vi "PositionToRollTatic.vi"(7 "Game in":refnum<class "Game.lvclass">, 8 "error in (no error)":errorcluster, 9 "first call":bool, 10 "Robot":refnum<class "Robot.lvclass">, 11 "PositionToRollTatic in":refnum<class "PositionToRollTatic.lvclass">) -> (0 "error out":errorcluster, 2 "Robot out":refnum<class "Robot.lvclass">, 3 "PositionToRollTatic out":refnum<class "PositionToRollTatic.lvclass">)   [LabVIEW 2018, in "PositionToRollTatic.lvclass"]
uses:
  PositionToRollTatic.lvclass
  Robot_class/Robot.lvclass
  Game_class/Game.lvclass
  Tactic_class/Tactic.lvclass/Tactic.ctl
  Robot_class/tactics.ctl
  Skillbook_class/Skillbook.lvclass/Skillbook.ctl
  Object_class/Object.lvclass/Object.ctl
  Robot_class/Robot.lvclass/Robot.ctl
  <vilib>/Analysis/_algsub.llb/Real Vector Norm.vi
  Skillbook_class/Read PositionToRollSkill.vi
  Object_class/Read x.vi
  Object_class/Read y.vi
  Robot_class/Read orientation.vi
  Robot_class/Read dest_x.vi
  Robot_class/Read dest_y.vi
  Robot_class/Read dest_orientation.vi
  Skillbook_class/Read HaltSkill.vi
  Tactic_class/Read Skillbook.vi
  Robot_class/Write tactic.vi
  Skillbook_class/Skillbook.lvclass
  PositionToRollSkill_class/PositionToRollSkill.lvclass
  HaltSkill_class/HaltSkill.lvclass
  <vilib>/Analysis/NI_AALPro.lvlib
panel:
  out "Sucsses":bool
  out "x .or. y?":bool
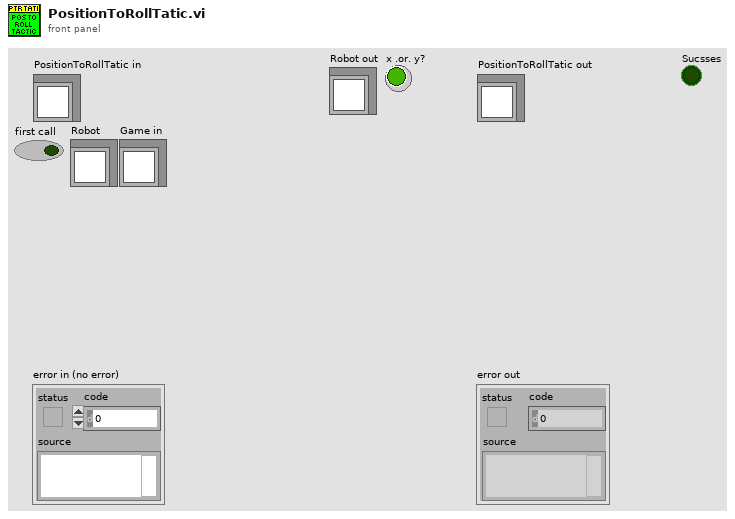
[diagram p1: front panel]
types:
  T1 = typedef "tactics.ctl" = enum16{"Roller", "PrepareRollToPassRollerGoTo", "PrepareRollToPassReceiverGoTo", "WaitRoll", "PositionToRoll", "PenaltyAttacker", "PassObserver", "PenaltyDefense", "Test", "DefendGoal", "Marker", "FollowAttacker", "DefendArea", "Shoot", "AttackerAimGoal", "AttackerBallOutOfField", "AttackerBlock", "AttackerStop", "Duelist", "Halt", "ZigZag", "GoTo", "Timeout", "KickToPassReceiver", "PositionToReceivePass", "PassReceiver", "WaitPass"}
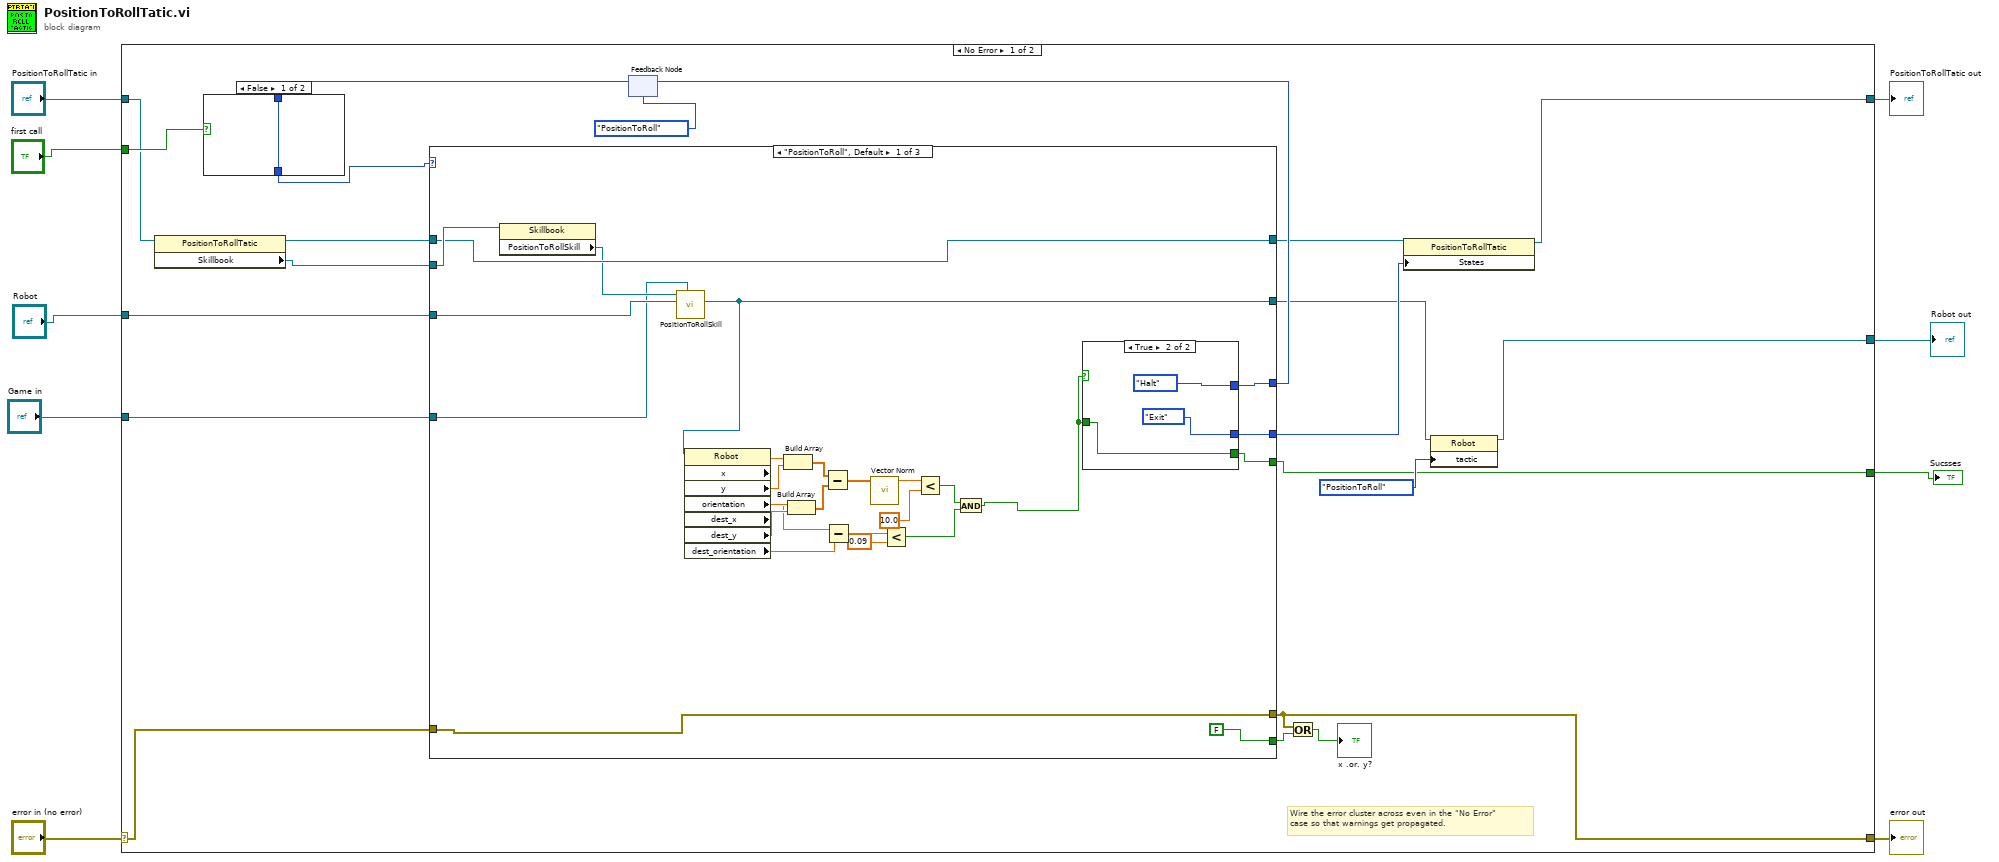
[diagram p0: block diagram]
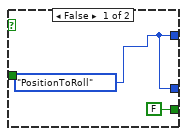
[diagram p2: hidden frame]
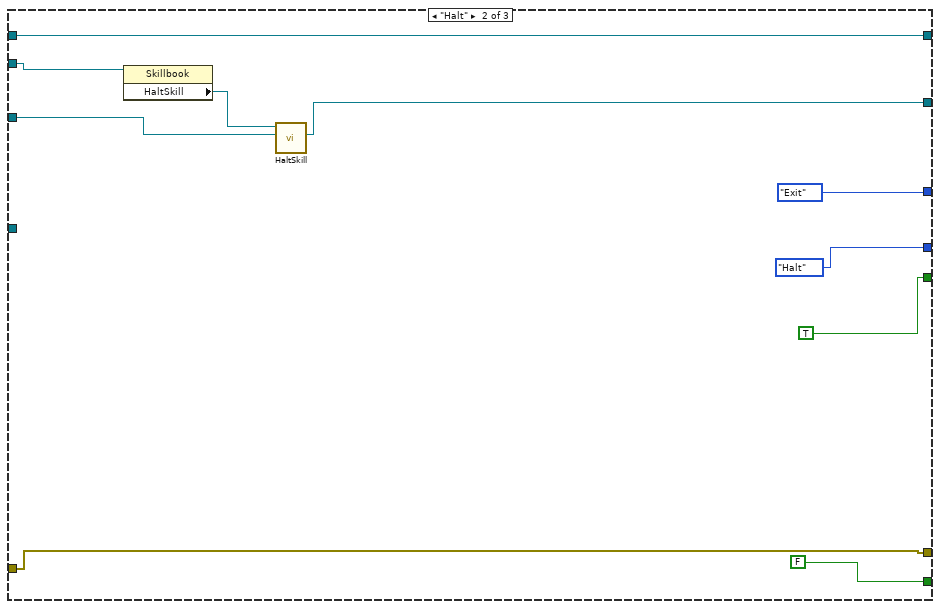
[diagram p3: hidden frame]
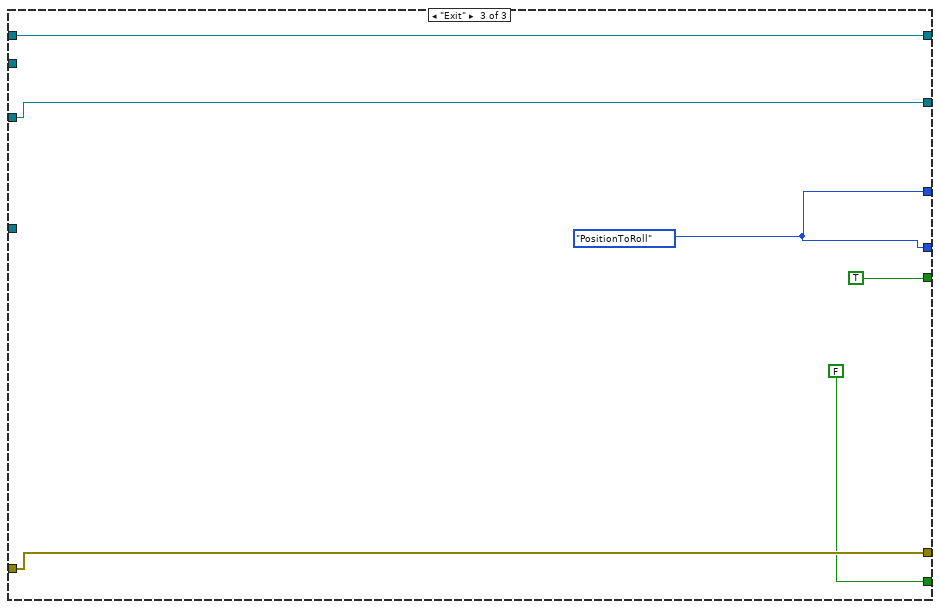
[diagram p4: hidden frame]
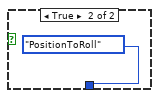
[diagram p5: hidden frame]
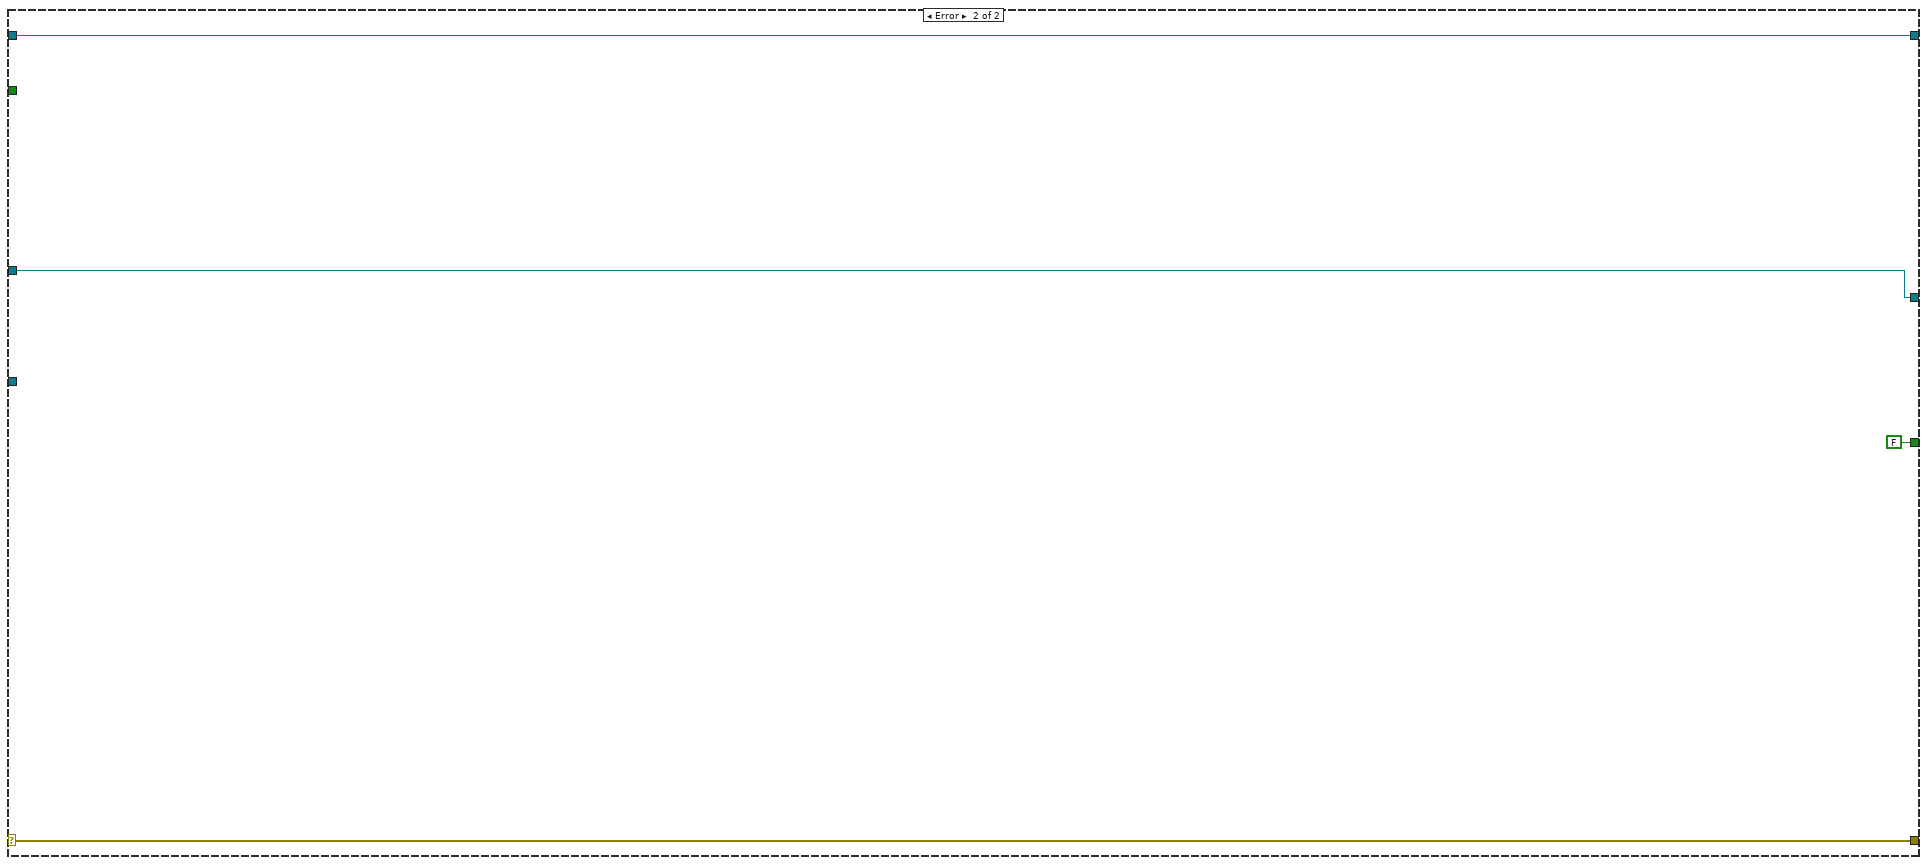
[diagram p6: hidden frame]
diagram:
  n1 = case shown="No Error" "error in (no error)" {
    selector: "error in (no error)" -> [w17 w84]
    tunnel: [w14 w84] -> w8
    tunnel: [w18 w83] -> w6
    tunnel: "PositionToRollTatic in" -> [w29 w83]
    tunnel: "first call" -> [w30 _]
    tunnel: "Robot" -> [w26 w82]
    tunnel: "Game in" -> [w25 _]
    tunnel: [w19 w82] -> w2
    tunnel: [w13 FALSE ("x .or. y?")] -> w1
    frame No Error {
      # "Wire the error cluster across even in the \"No Error\"\ncase so that warnings get propagated."
      n2 = property class="PositionToRollTatic"(reference=w29) -> (reference out=w27:refnum<class "PositionToRollTatic.lvclass">, "Skillbook"=w28:refnum<class "Skillbook.lvclass">)  [unwired: 1 in, 1 out]
      n3 = feedback #1(enum16{"PositionToRoll", "Halt", "Exit"}."PositionToRoll" ("States")) -> (w23:enum16{"PositionToRoll", "Halt", "Exit"})
      n4 = case shown="False" w30 {
        tunnel: [w79 enum16{"PositionToRoll", "Halt", "Exit"}."PositionToRoll" ("States")] -> w10
        tunnel: w23 -> [w79 _]
        frame False {
        }
        frame True {
        }
      }
      n5 = case shown="\"PositionToRoll\", Default" w10 {
        tunnel: w28 -> [w57 w72 _]
        tunnel: w27 -> [w56 w68 w78]
        tunnel: [w56 w68 w78] -> w12
        tunnel: w26 -> [w54 w69 w77]
        tunnel: w25 -> [w53 _ _]
        tunnel: [w52 enum16{"PositionToRoll", "Halt", "Exit"}."Exit" ("States") w73] -> w24
        tunnel: [w51 enum16{"PositionToRoll", "Halt", "Exit"}."Halt" ("States") w73] -> w22
        tunnel: [w34 w70 w77] -> w21
        tunnel: [FALSE ("x .or. y?") FALSE ("x .or. y?") FALSE ("x .or. y?")] -> w16
        tunnel: w17 -> [w31 w63 w76]
        tunnel: [w31 w63 w76] -> w14
        tunnel: [w33 TRUE ("x .or. y?") TRUE ("x .or. y?")] -> w13
        frame "PositionToRoll", Default {
          n6 = property class="Skillbook"(reference=w57) -> ("PositionToRollSkill"=w55:refnum<class "PositionToRollSkill.lvclass">)  [unwired: 1 in, 2 out]
          n7 = call "PositionToRollSkill.vi"("Game in"=w53, "Robot"=w54, "PositionToRollSkill in"=w55) -> ("Robot out"=w34:refnum<class "Robot.lvclass">)  [unwired: 6 in, 2 out]
          n8 = property class="Robot"(reference=w34) -> ("x"=w49:dbl, "y"=w48:dbl, "orientation"=w43:dbl, "dest_x"=w47:dbl, "dest_y"=w46:dbl, "dest_orientation"=w42:dbl)  [unwired: 1 in, 2 out]
          n9 = Build Array(w49, w48) -> (w45:dbl[])
          n10 = Build Array(w47, w46) -> (w44:dbl[])
          n11 = Subtract(x=w45, y=w44) -> (x-y=w41:dbl[])
          n12 = Subtract(x=w43, y=w42) -> (x-y=w38:dbl)
          n13 = call-poly <vilib>:"Vector Norm.vi"("Input Vector"=w41) -> ("norm"=w40:dbl)  [unwired: 9 in, 1 out]
          n14 = Less?(x=w38, y=0.09) -> (x < y?=w35:bool)
          n15 = Less?(x=w40, y=10.0) -> (x < y?=w36:bool)
          n16 = And(x=w36, y=w35) -> (x .and. y?=w32:bool)
          n17 = case shown="True" w32 {
            tunnel: [w58 enum16{"PositionToRoll", "Halt", "Exit"}."Halt" ("States")] -> w52
            tunnel: [w58 enum16{"PositionToRoll", "Halt", "Exit"}."Exit" ("States")] -> w51
            tunnel: w32 -> [_ w62]
            tunnel: [FALSE w62] -> w33
            frame False {
              w58 = enum16{"PositionToRoll", "Halt", "Exit"}."PositionToRoll" ("States")
            }
            frame True {
            }
          }
        }
        frame "Halt" {
          n18 = property class="Skillbook"(reference=w72) -> ("HaltSkill"=w71:refnum<class "HaltSkill.lvclass">)  [unwired: 1 in, 2 out]
          n19 = call-dynamic "HaltSkill.vi"("Robot"=w69, "HaltSkill in"=w71) -> ("Robot out"=w70:refnum<class "Robot.lvclass">)  [unwired: 7 in, 2 out]
        }
        frame "Exit" {
          w73 = enum16{"PositionToRoll", "Halt", "Exit"}."PositionToRoll" ("States")
        }
      }
      n20 = feedback-in #1(w24) -> ()
      n21 = Or(x=w14, y=w16) -> (x .or. y?=→"x .or. y?":bool)
      n22 = property class="PositionToRollTatic"(reference=w12, "States"=w22) -> (reference out=w18:refnum<class "PositionToRollTatic.lvclass">)  [unwired: 1 in, 1 out]
      n23 = property class="Robot"(reference=w21, "tactic"=tactics."PositionToRoll") -> (reference out=w19:refnum<class "Robot.lvclass">)  [unwired: 1 in, 1 out]
    }
    frame Error {
    }
  }
  "error out" <- w8
  "PositionToRollTatic out" <- w6
  "Robot out" <- w2
  "Sucsses" <- w1
